vi "NaCTA_configure.vi"() -> ()   [LabVIEW 2020]
uses:
  Instrument drivers/Arduino/ctls_and_globals/Arduino tx msg cluster.ctl
panel:
  in  "a4":dbl=1.0
  in  "a3":dbl=1.0
  in  "Enable USB stream":bool=TRUE
  in  "a2":dbl=1.0
  in  "T0 offset (deg C)":dbl
  in  "P_atmos offset (Pa)":dbl
  in  "Port":refnum<visa-resource-name>
  in  "Get / Set":u8(ring) items=["Get", "Set"]
  in  "a1":dbl=1.0
  in  "a0":dbl=1.0
  out "Read-back":string
  out "Status comment":string
  in  "Address":u8=1
  # "Use this vi to configure the NaCTA 'hot-thermistor' node\nThese settings are retained in EEPROM and recalled on power-up."
  # "PN 05/02/2017"
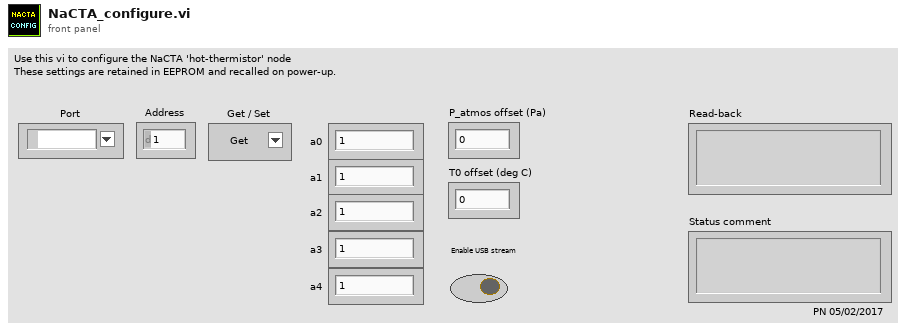
[diagram p1: front panel]
types:
  T1 = typedef "Arduino tx msg cluster.ctl" = cluster{"dest":u8, "A/D/C/I":string, "R/W":string, "chan":u8, "val (float)":sgl}
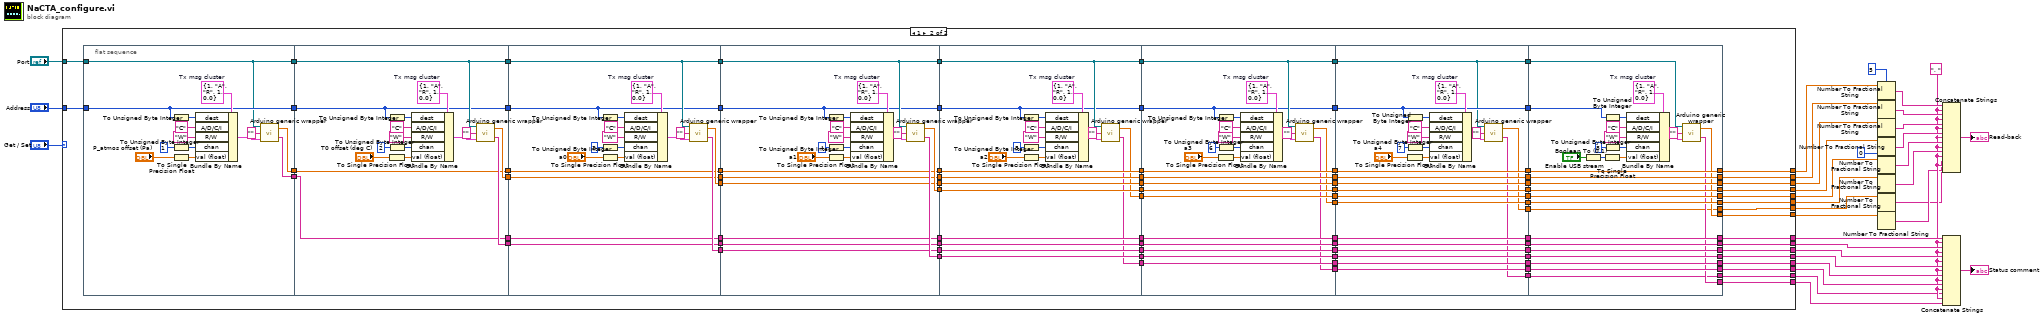
[diagram p0: block diagram]
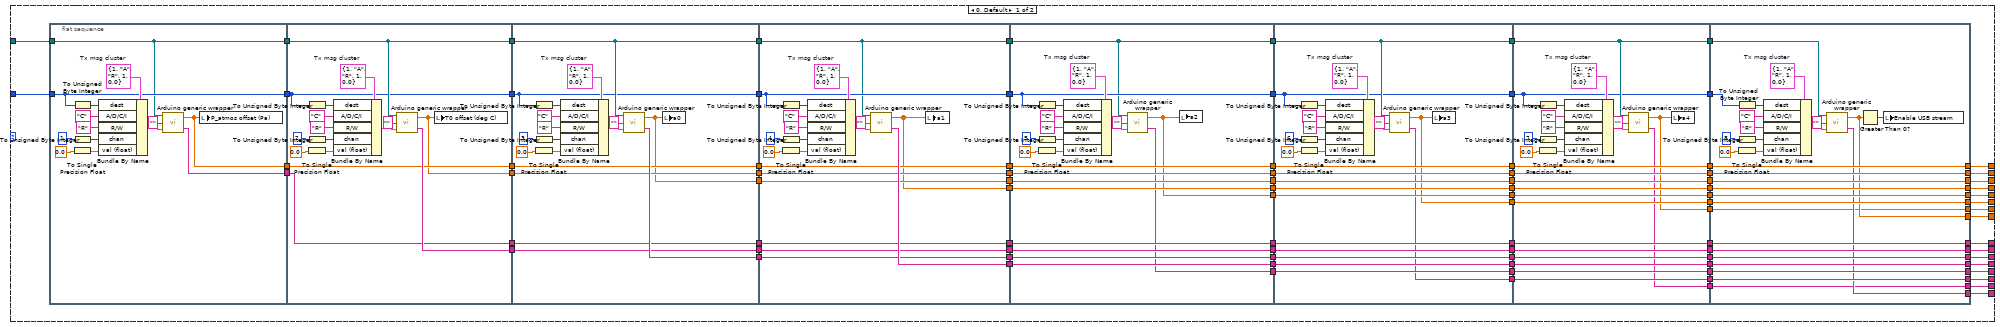
[diagram p2: hidden frame]
diagram:
  w4 = i16 5 ("precision (6)")
  w6 = ", "
  n1 = case shown="1" "Get / Set" {
    tunnel: "Address" -> [w101 w359]
    tunnel: [w93 w358] -> w27
    tunnel: [w97 w357] -> w26
    tunnel: [w98 w356] -> w24
    tunnel: [w94 w355] -> w23
    tunnel: [w95 w354] -> w22
    tunnel: [w96 w353] -> w21
    tunnel: [w99 w352] -> w20
    tunnel: [w100 w351] -> w19
    tunnel: "Port" -> [w102 w350]
    tunnel: [w70 w339] -> w12
    tunnel: [w67 w325] -> w11
    tunnel: [w65 w323] -> w7
    tunnel: [w69 w338] -> w10
    tunnel: [w68 w324] -> w9
    tunnel: [w66 w322] -> w8
    tunnel: [w34 w293] -> w2
    tunnel: [w33 w290] -> w1
    frame 0, Default {
      n2 = flat-sequence {
        tunnel: w101 -> [w126]
        tunnel: w102 -> [w125]
        tunnel: [w125] -> w120
        tunnel: [w126] -> w119
        tunnel: [w122] -> w118
        tunnel: [w124] -> w117
        tunnel: [w142] -> w116
        tunnel: [w141] -> w115
        tunnel: [w140] -> w114
        tunnel: [w136] -> w113
        tunnel: w120 -> [w142]
        tunnel: w119 -> [w141]
        tunnel: w118 -> [w138]
        tunnel: w117 -> [w139]
        tunnel: [w139] -> w112
        tunnel: [w138] -> w111
        tunnel: w116 -> [w160]
        tunnel: [w160] -> w110
        tunnel: w115 -> [w159]
        tunnel: [w159] -> w109
        tunnel: w114 -> [w157]
        tunnel: w113 -> [w155]
        tunnel: [w158] -> w108
        tunnel: [w152] -> w107
        tunnel: [w157] -> w106
        tunnel: [w156] -> w105
        tunnel: w112 -> [w156]
        tunnel: [w155] -> w104
        tunnel: [w154] -> w103
        tunnel: w111 -> [w154]
        tunnel: w110 -> [w171]
        tunnel: w109 -> [w172]
        tunnel: w108 -> [w178]
        tunnel: w107 -> [w179]
        tunnel: w106 -> [w177]
        tunnel: w105 -> [w176]
        tunnel: w104 -> [w175]
        tunnel: w103 -> [w174]
        tunnel: [w180] -> w92
        tunnel: [w170] -> w91
        tunnel: [w179] -> w90
        tunnel: [w178] -> w89
        tunnel: [w177] -> w88
        tunnel: [w176] -> w87
        tunnel: [w175] -> w86
        tunnel: [w174] -> w85
        tunnel: [w172] -> w76
        tunnel: [w171] -> w75
        tunnel: w92 -> [w210]
        tunnel: w91 -> [w209]
        tunnel: w90 -> [w208]
        tunnel: w89 -> [w207]
        tunnel: w88 -> [w206]
        tunnel: w87 -> [w205]
        tunnel: w86 -> [w204]
        tunnel: w85 -> [w203]
        tunnel: [w210] -> w84
        tunnel: [w209] -> w83
        tunnel: [w208] -> w82
        tunnel: [w207] -> w81
        tunnel: [w206] -> w80
        tunnel: [w205] -> w79
        tunnel: [w204] -> w78
        tunnel: [w203] -> w77
        tunnel: w76 -> [w193]
        tunnel: w75 -> [w192]
        tunnel: [w193] -> w74
        tunnel: [w192] -> w73
        tunnel: [w191] -> w72
        tunnel: [w190] -> w71
        tunnel: w84 -> [w234]
        tunnel: w83 -> [w233]
        tunnel: w82 -> [w232]
        tunnel: w81 -> [w231]
        tunnel: w80 -> [w230]
        tunnel: w79 -> [w229]
        tunnel: w78 -> [w228]
        tunnel: w77 -> [w227]
        tunnel: [w234] -> w64
        tunnel: [w233] -> w62
        tunnel: [w232] -> w60
        tunnel: [w231] -> w58
        tunnel: [w230] -> w56
        tunnel: [w229] -> w54
        tunnel: [w228] -> w52
        tunnel: [w227] -> w50
        tunnel: w74 -> [w214]
        tunnel: w73 -> [w215]
        tunnel: [w214] -> w48
        tunnel: [w215] -> w46
        tunnel: w72 -> [w226]
        tunnel: w71 -> [w225]
        tunnel: [w226] -> w44
        tunnel: [w225] -> w42
        tunnel: [w212] -> w40
        tunnel: [w213] -> w38
        tunnel: w64 -> [w260]
        tunnel: [w260] -> w63
        tunnel: w62 -> [w259]
        tunnel: [w259] -> w61
        tunnel: w60 -> [w258]
        tunnel: [w258] -> w59
        tunnel: w58 -> [w257]
        tunnel: [w257] -> w57
        tunnel: w56 -> [w256]
        tunnel: [w256] -> w55
        tunnel: w54 -> [w255]
        tunnel: [w255] -> w53
        tunnel: w52 -> [w254]
        tunnel: [w254] -> w51
        tunnel: w50 -> [w253]
        tunnel: [w253] -> w49
        tunnel: w48 -> [w236]
        tunnel: [w236] -> w47
        tunnel: w46 -> [w239]
        tunnel: [w239] -> w45
        tunnel: w44 -> [w252]
        tunnel: [w252] -> w43
        tunnel: w42 -> [w251]
        tunnel: [w251] -> w41
        tunnel: w40 -> [w250]
        tunnel: [w250] -> w39
        tunnel: w38 -> [w249]
        tunnel: [w249] -> w37
        tunnel: [w238] -> w36
        tunnel: [w237] -> w35
        tunnel: w63 -> [w289]
        tunnel: w61 -> [w288]
        tunnel: w59 -> [w287]
        tunnel: w57 -> [w286]
        tunnel: w55 -> [w285]
        tunnel: w53 -> [w284]
        tunnel: w51 -> [w283]
        tunnel: w49 -> [w282]
        tunnel: w47 -> [w267]
        tunnel: w45 -> [w266]
        tunnel: w43 -> [w281]
        tunnel: w41 -> [w280]
        tunnel: w39 -> [w279]
        tunnel: w37 -> [w278]
        tunnel: [w268] -> w65
        tunnel: [w264] -> w66
        tunnel: [w278] -> w67
        tunnel: [w279] -> w68
        tunnel: [w280] -> w69
        tunnel: [w281] -> w70
        tunnel: [w282] -> w100
        tunnel: [w283] -> w99
        tunnel: [w284] -> w96
        tunnel: [w285] -> w95
        tunnel: [w286] -> w94
        tunnel: [w287] -> w98
        tunnel: [w288] -> w97
        tunnel: [w289] -> w93
        tunnel: w36 -> [w263]
        tunnel: w35 -> [w262]
        tunnel: [w263] -> w34
        tunnel: [w262] -> w33
        frame #0 {
          w134 = T1 {"dest"=1, "A/D/C/I"="A", "R/W"="R", "chan"=1, "val (float)"=0.0}  # Tx msg cluster
          n3 = To Unsigned Byte Integer(number=w126) -> (unsigned 8bit integer=w132:u8)
          n4 = To Unsigned Byte Integer(number=u8 1) -> (unsigned 8bit integer=w133:u8)
          n5 = To Single Precision Float(number=0.0) -> (single precision float=w130:sgl)
          n6 = Bundle By Name(cluster=w134, "dest"=w132, "A/D/C/I"="C" ("A/D"), "R/W"="R", "chan"=w133, "val (float)"=w130) -> (w131:T1)
          n7 = call "Arduino generic wrapper.vi"("Tx msg cluster"=w131, "Channel Name"="", "Port name"=w125) -> ("Scan comment"=w124:string, "Output"=w122:dbl)
          n8 = local write "P_atmos offset (Pa)"(w122) -> ()
        }
        frame #1 {
          w143 = T1 {"dest"=1, "A/D/C/I"="A", "R/W"="R", "chan"=1, "val (float)"=0.0}  # Tx msg cluster
          n9 = To Unsigned Byte Integer(number=w141) -> (unsigned 8bit integer=w145:u8)
          n10 = To Unsigned Byte Integer(number=u8 2) -> (unsigned 8bit integer=w144:u8)
          n11 = To Single Precision Float(number=0.0) -> (single precision float=w147:sgl)
          n12 = Bundle By Name(cluster=w143, "dest"=w145, "A/D/C/I"="C" ("A/D"), "R/W"="R", "chan"=w144, "val (float)"=w147) -> (w146:T1)
          n13 = call "Arduino generic wrapper.vi"("Tx msg cluster"=w146, "Channel Name"="", "Port name"=w142) -> ("Scan comment"=w140:string, "Output"=w136:dbl)
          n14 = local write "T0 offset (deg C)"(w136) -> ()
        }
        frame #2 {
          w168 = T1 {"dest"=1, "A/D/C/I"="A", "R/W"="R", "chan"=1, "val (float)"=0.0}  # Tx msg cluster
          n15 = To Unsigned Byte Integer(number=w159) -> (unsigned 8bit integer=w166:u8)
          n16 = To Unsigned Byte Integer(number=u8 3) -> (unsigned 8bit integer=w167:u8)
          n17 = To Single Precision Float(number=0.0) -> (single precision float=w164:sgl)
          n18 = Bundle By Name(cluster=w168, "dest"=w166, "A/D/C/I"="C" ("A/D"), "R/W"="R", "chan"=w167, "val (float)"=w164) -> (w165:T1)
          n19 = call "Arduino generic wrapper.vi"("Tx msg cluster"=w165, "Channel Name"="", "Port name"=w160) -> ("Scan comment"=w158:string, "Output"=w152:dbl)
          n20 = local write "a0"(w152) -> ()
        }
        frame #3 {
          w187 = T1 {"dest"=1, "A/D/C/I"="A", "R/W"="R", "chan"=1, "val (float)"=0.0}  # Tx msg cluster
          n21 = To Unsigned Byte Integer(number=w172) -> (unsigned 8bit integer=w181:u8)
          n22 = To Unsigned Byte Integer(number=u8 4) -> (unsigned 8bit integer=w182:u8)
          n23 = To Single Precision Float(number=0.0) -> (single precision float=w184:sgl)
          n24 = Bundle By Name(cluster=w187, "dest"=w181, "A/D/C/I"="C" ("A/D"), "R/W"="R", "chan"=w182, "val (float)"=w184) -> (w183:T1)
          n25 = call "Arduino generic wrapper.vi"("Tx msg cluster"=w183, "Channel Name"="", "Port name"=w171) -> ("Scan comment"=w180:string, "Output"=w170:dbl)
          n26 = local write "a1"(w170) -> ()
        }
        frame #4 {
          w195 = T1 {"dest"=1, "A/D/C/I"="A", "R/W"="R", "chan"=1, "val (float)"=0.0}  # Tx msg cluster
          n27 = To Unsigned Byte Integer(number=w193) -> (unsigned 8bit integer=w201:u8)
          n28 = To Unsigned Byte Integer(number=u8 5) -> (unsigned 8bit integer=w200:u8)
          n29 = To Single Precision Float(number=0.0) -> (single precision float=w198:sgl)
          n30 = Bundle By Name(cluster=w195, "dest"=w201, "A/D/C/I"="C" ("A/D"), "R/W"="R", "chan"=w200, "val (float)"=w198) -> (w199:T1)
          n31 = call "Arduino generic wrapper.vi"("Tx msg cluster"=w199, "Channel Name"="", "Port name"=w192) -> ("Scan comment"=w191:string, "Output"=w190:dbl)
          n32 = local write "a2"(w190) -> ()
        }
        frame #5 {
          w223 = T1 {"dest"=1, "A/D/C/I"="A", "R/W"="R", "chan"=1, "val (float)"=0.0}  # Tx msg cluster
          n33 = To Unsigned Byte Integer(number=w214) -> (unsigned 8bit integer=w217:u8)
          n34 = To Unsigned Byte Integer(number=u8 6) -> (unsigned 8bit integer=w218:u8)
          n35 = To Single Precision Float(number=0.0) -> (single precision float=w220:sgl)
          n36 = Bundle By Name(cluster=w223, "dest"=w217, "A/D/C/I"="C" ("A/D"), "R/W"="R", "chan"=w218, "val (float)"=w220) -> (w219:T1)
          n37 = call "Arduino generic wrapper.vi"("Tx msg cluster"=w219, "Channel Name"="", "Port name"=w215) -> ("Scan comment"=w213:string, "Output"=w212:dbl)
          n38 = local write "a3"(w212) -> ()
        }
        frame #6 {
          w241 = T1 {"dest"=1, "A/D/C/I"="A", "R/W"="R", "chan"=1, "val (float)"=0.0}  # Tx msg cluster
          n39 = To Unsigned Byte Integer(number=w236) -> (unsigned 8bit integer=w247:u8)
          n40 = To Unsigned Byte Integer(number=u8 7) -> (unsigned 8bit integer=w246:u8)
          n41 = To Single Precision Float(number=0.0) -> (single precision float=w244:sgl)
          n42 = Bundle By Name(cluster=w241, "dest"=w247, "A/D/C/I"="C" ("A/D"), "R/W"="R", "chan"=w246, "val (float)"=w244) -> (w245:T1)
          n43 = call "Arduino generic wrapper.vi"("Tx msg cluster"=w245, "Channel Name"="", "Port name"=w239) -> ("Scan comment"=w237:string, "Output"=w238:dbl)
          n44 = local write "a4"(w238) -> ()
        }
        frame #7 {
          w270 = T1 {"dest"=1, "A/D/C/I"="A", "R/W"="R", "chan"=1, "val (float)"=0.0}  # Tx msg cluster
          n45 = To Unsigned Byte Integer(number=w267) -> (unsigned 8bit integer=w276:u8)
          n46 = To Unsigned Byte Integer(number=u8 8) -> (unsigned 8bit integer=w275:u8)
          n47 = To Single Precision Float(number=0.0) -> (single precision float=w273:sgl)
          n48 = Bundle By Name(cluster=w270, "dest"=w276, "A/D/C/I"="C" ("A/D"), "R/W"="R", "chan"=w275, "val (float)"=w273) -> (w274:T1)
          n49 = call "Arduino generic wrapper.vi"("Tx msg cluster"=w274, "Channel Name"="", "Port name"=w266) -> ("Scan comment"=w268:string, "Output"=w264:dbl)
          n50 = Greater Than 0?(x=w264) -> (x > 0?=w265:bool)
          n51 = local write "Enable USB stream"(w265) -> ()
        }
      }
    }
    frame 1 {
      n52 = flat-sequence {
        tunnel: w359 -> [w383]
        tunnel: w350 -> [w382]
        tunnel: [w382] -> w377
        tunnel: [w383] -> w376
        tunnel: [w381] -> w375
        tunnel: [w380] -> w374
        tunnel: [w399] -> w373
        tunnel: [w398] -> w372
        tunnel: [w397] -> w371
        tunnel: [w396] -> w370
        tunnel: w377 -> [w399]
        tunnel: w376 -> [w398]
        tunnel: w375 -> [w394]
        tunnel: w374 -> [w395]
        tunnel: [w395] -> w369
        tunnel: [w394] -> w368
        tunnel: w373 -> [w417]
        tunnel: [w417] -> w367
        tunnel: w372 -> [w416]
        tunnel: [w416] -> w366
        tunnel: w371 -> [w413]
        tunnel: w370 -> [w411]
        tunnel: [w415] -> w365
        tunnel: [w414] -> w364
        tunnel: [w413] -> w363
        tunnel: [w412] -> w362
        tunnel: w369 -> [w412]
        tunnel: [w411] -> w361
        tunnel: [w410] -> w360
        tunnel: w368 -> [w410]
        tunnel: w367 -> [w429]
        tunnel: w366 -> [w428]
        tunnel: w365 -> [w434]
        tunnel: w364 -> [w435]
        tunnel: w363 -> [w433]
        tunnel: w362 -> [w432]
        tunnel: w361 -> [w431]
        tunnel: w360 -> [w430]
        tunnel: [w437] -> w349
        tunnel: [w436] -> w348
        tunnel: [w435] -> w347
        tunnel: [w434] -> w346
        tunnel: [w433] -> w345
        tunnel: [w432] -> w344
        tunnel: [w431] -> w343
        tunnel: [w430] -> w342
        tunnel: [w429] -> w341
        tunnel: [w428] -> w340
        tunnel: w349 -> [w467]
        tunnel: w348 -> [w466]
        tunnel: w347 -> [w465]
        tunnel: w346 -> [w464]
        tunnel: w345 -> [w463]
        tunnel: w344 -> [w462]
        tunnel: w343 -> [w461]
        tunnel: w342 -> [w460]
        tunnel: w341 -> [w449]
        tunnel: w340 -> [w448]
        tunnel: [w467] -> w337
        tunnel: [w466] -> w336
        tunnel: [w465] -> w335
        tunnel: [w464] -> w334
        tunnel: [w463] -> w333
        tunnel: [w462] -> w332
        tunnel: [w461] -> w331
        tunnel: [w460] -> w330
        tunnel: [w451] -> w329
        tunnel: [w450] -> w328
        tunnel: [w449] -> w327
        tunnel: [w448] -> w326
        tunnel: w337 -> [w491]
        tunnel: w336 -> [w490]
        tunnel: w335 -> [w489]
        tunnel: w334 -> [w488]
        tunnel: w333 -> [w487]
        tunnel: w332 -> [w486]
        tunnel: w331 -> [w485]
        tunnel: w330 -> [w484]
        tunnel: w329 -> [w483]
        tunnel: w328 -> [w482]
        tunnel: w327 -> [w471]
        tunnel: w326 -> [w470]
        tunnel: [w491] -> w321
        tunnel: [w490] -> w319
        tunnel: [w489] -> w317
        tunnel: [w488] -> w315
        tunnel: [w487] -> w313
        tunnel: [w486] -> w311
        tunnel: [w485] -> w309
        tunnel: [w484] -> w307
        tunnel: [w483] -> w305
        tunnel: [w482] -> w303
        tunnel: [w473] -> w301
        tunnel: [w472] -> w299
        tunnel: [w471] -> w297
        tunnel: [w470] -> w295
        tunnel: w321 -> [w517]
        tunnel: [w517] -> w320
        tunnel: w319 -> [w516]
        tunnel: [w516] -> w318
        tunnel: w317 -> [w515]
        tunnel: [w515] -> w316
        tunnel: w315 -> [w514]
        tunnel: [w514] -> w314
        tunnel: w313 -> [w513]
        tunnel: [w513] -> w312
        tunnel: w311 -> [w512]
        tunnel: [w512] -> w310
        tunnel: w309 -> [w511]
        tunnel: [w511] -> w308
        tunnel: w307 -> [w510]
        tunnel: [w510] -> w306
        tunnel: w305 -> [w509]
        tunnel: [w509] -> w304
        tunnel: w303 -> [w508]
        tunnel: [w508] -> w302
        tunnel: w301 -> [w507]
        tunnel: [w507] -> w300
        tunnel: w299 -> [w506]
        tunnel: [w506] -> w298
        tunnel: w297 -> [w495]
        tunnel: [w495] -> w296
        tunnel: w295 -> [w496]
        tunnel: [w496] -> w294
        tunnel: [w494] -> w292
        tunnel: [w493] -> w291
        tunnel: w320 -> [w546]
        tunnel: w318 -> [w545]
        tunnel: w316 -> [w544]
        tunnel: w314 -> [w543]
        tunnel: w312 -> [w542]
        tunnel: w310 -> [w541]
        tunnel: w308 -> [w540]
        tunnel: w306 -> [w539]
        tunnel: w304 -> [w538]
        tunnel: w302 -> [w537]
        tunnel: w300 -> [w536]
        tunnel: w298 -> [w535]
        tunnel: w296 -> [w523]
        tunnel: w294 -> [w524]
        tunnel: [w525] -> w322
        tunnel: [w526] -> w323
        tunnel: [w535] -> w324
        tunnel: [w536] -> w325
        tunnel: [w537] -> w338
        tunnel: [w538] -> w339
        tunnel: [w539] -> w351
        tunnel: [w540] -> w352
        tunnel: [w541] -> w353
        tunnel: [w542] -> w354
        tunnel: [w543] -> w355
        tunnel: [w544] -> w356
        tunnel: [w545] -> w357
        tunnel: [w546] -> w358
        tunnel: [w520] -> w293
        tunnel: w292 -> [w520]
        tunnel: w291 -> [w519]
        tunnel: [w519] -> w290
        frame #0 {
          w391 = T1 {"dest"=1, "A/D/C/I"="A", "R/W"="R", "chan"=1, "val (float)"=0.0}  # Tx msg cluster
          n53 = To Unsigned Byte Integer(number=w383) -> (unsigned 8bit integer=w389:u8)
          n54 = To Unsigned Byte Integer(number=u8 1) -> (unsigned 8bit integer=w390:u8)
          n55 = To Single Precision Float(number="P_atmos offset (Pa)") -> (single precision float=w387:sgl)
          n56 = Bundle By Name(cluster=w391, "dest"=w389, "A/D/C/I"="C" ("A/D"), "R/W"="W", "chan"=w390, "val (float)"=w387) -> (w388:T1)
          n57 = call "Arduino generic wrapper.vi"("Tx msg cluster"=w388, "Channel Name"="", "Port name"=w382) -> ("Scan comment"=w380:string, "Output"=w381:dbl)
        }
        frame #1 {
          w400 = T1 {"dest"=1, "A/D/C/I"="A", "R/W"="R", "chan"=1, "val (float)"=0.0}  # Tx msg cluster
          n58 = To Unsigned Byte Integer(number=w398) -> (unsigned 8bit integer=w402:u8)
          n59 = To Unsigned Byte Integer(number=u8 2) -> (unsigned 8bit integer=w401:u8)
          n60 = To Single Precision Float(number="T0 offset (deg C)") -> (single precision float=w404:sgl)
          n61 = Bundle By Name(cluster=w400, "dest"=w402, "A/D/C/I"="C" ("A/D"), "R/W"="W", "chan"=w401, "val (float)"=w404) -> (w403:T1)
          n62 = call "Arduino generic wrapper.vi"("Tx msg cluster"=w403, "Channel Name"="", "Port name"=w399) -> ("Scan comment"=w397:string, "Output"=w396:dbl)
        }
        frame #2 {
          w425 = T1 {"dest"=1, "A/D/C/I"="A", "R/W"="R", "chan"=1, "val (float)"=0.0}  # Tx msg cluster
          n63 = To Unsigned Byte Integer(number=w416) -> (unsigned 8bit integer=w423:u8)
          n64 = To Unsigned Byte Integer(number=u8 3) -> (unsigned 8bit integer=w424:u8)
          n65 = To Single Precision Float(number="a0") -> (single precision float=w421:sgl)
          n66 = Bundle By Name(cluster=w425, "dest"=w423, "A/D/C/I"="C" ("A/D"), "R/W"="W", "chan"=w424, "val (float)"=w421) -> (w422:T1)
          n67 = call "Arduino generic wrapper.vi"("Tx msg cluster"=w422, "Channel Name"="", "Port name"=w417) -> ("Scan comment"=w415:string, "Output"=w414:dbl)
        }
        frame #3 {
          w444 = T1 {"dest"=1, "A/D/C/I"="A", "R/W"="R", "chan"=1, "val (float)"=0.0}  # Tx msg cluster
          n68 = To Unsigned Byte Integer(number=w428) -> (unsigned 8bit integer=w438:u8)
          n69 = To Unsigned Byte Integer(number=u8 4) -> (unsigned 8bit integer=w439:u8)
          n70 = To Single Precision Float(number="a1") -> (single precision float=w441:sgl)
          n71 = Bundle By Name(cluster=w444, "dest"=w438, "A/D/C/I"="C" ("A/D"), "R/W"="W", "chan"=w439, "val (float)"=w441) -> (w440:T1)
          n72 = call "Arduino generic wrapper.vi"("Tx msg cluster"=w440, "Channel Name"="", "Port name"=w429) -> ("Scan comment"=w437:string, "Output"=w436:dbl)
        }
        frame #4 {
          w453 = T1 {"dest"=1, "A/D/C/I"="A", "R/W"="R", "chan"=1, "val (float)"=0.0}  # Tx msg cluster
          n73 = To Unsigned Byte Integer(number=w448) -> (unsigned 8bit integer=w459:u8)
          n74 = To Unsigned Byte Integer(number=u8 5) -> (unsigned 8bit integer=w458:u8)
          n75 = To Single Precision Float(number="a2") -> (single precision float=w456:sgl)
          n76 = Bundle By Name(cluster=w453, "dest"=w459, "A/D/C/I"="C" ("A/D"), "R/W"="W", "chan"=w458, "val (float)"=w456) -> (w457:T1)
          n77 = call "Arduino generic wrapper.vi"("Tx msg cluster"=w457, "Channel Name"="", "Port name"=w449) -> ("Scan comment"=w451:string, "Output"=w450:dbl)
        }
        frame #5 {
          w480 = T1 {"dest"=1, "A/D/C/I"="A", "R/W"="R", "chan"=1, "val (float)"=0.0}  # Tx msg cluster
          n78 = To Unsigned Byte Integer(number=w470) -> (unsigned 8bit integer=w474:u8)
          n79 = To Unsigned Byte Integer(number=u8 6) -> (unsigned 8bit integer=w475:u8)
          n80 = To Single Precision Float(number="a3") -> (single precision float=w477:sgl)
          n81 = Bundle By Name(cluster=w480, "dest"=w474, "A/D/C/I"="C" ("A/D"), "R/W"="W", "chan"=w475, "val (float)"=w477) -> (w476:T1)
          n82 = call "Arduino generic wrapper.vi"("Tx msg cluster"=w476, "Channel Name"="", "Port name"=w471) -> ("Scan comment"=w473:string, "Output"=w472:dbl)
        }
        frame #6 {
          w499 = T1 {"dest"=1, "A/D/C/I"="A", "R/W"="R", "chan"=1, "val (float)"=0.0}  # Tx msg cluster
          n83 = To Unsigned Byte Integer(number=w496) -> (unsigned 8bit integer=w505:u8)
          n84 = To Unsigned Byte Integer(number=u8 7) -> (unsigned 8bit integer=w504:u8)
          n85 = To Single Precision Float(number="a4") -> (single precision float=w502:sgl)
          n86 = Bundle By Name(cluster=w499, "dest"=w505, "A/D/C/I"="C" ("A/D"), "R/W"="W", "chan"=w504, "val (float)"=w502) -> (w503:T1)
          n87 = call "Arduino generic wrapper.vi"("Tx msg cluster"=w503, "Channel Name"="", "Port name"=w495) -> ("Scan comment"=w493:string, "Output"=w494:dbl)
        }
        frame #7 {
          w528 = T1 {"dest"=1, "A/D/C/I"="A", "R/W"="R", "chan"=1, "val (float)"=0.0}  # Tx msg cluster
          n88 = Boolean To (0,1)(Boolean="Enable USB stream") -> (0, 1=w522:i16)
          n89 = To Unsigned Byte Integer(number=w524) -> (unsigned 8bit integer=w534:u8)
          n90 = To Unsigned Byte Integer(number=u8 8) -> (unsigned 8bit integer=w533:u8)
          n91 = To Single Precision Float(number=w522) -> (single precision float=w531:sgl)
          n92 = Bundle By Name(cluster=w528, "dest"=w534, "A/D/C/I"="C" ("A/D"), "R/W"="W", "chan"=w533, "val (float)"=w531) -> (w532:T1)
          n93 = call "Arduino generic wrapper.vi"("Tx msg cluster"=w532, "Channel Name"="", "Port name"=w523) -> ("Scan comment"=w526:string, "Output"=w525:dbl)
        }
      }
    }
  }
  n94 = Number To Fractional String(number=w19, precision (6)=w4) -> (F-format string=w31:string)  [unwired: 2 in]
  n95 = Number To Fractional String(number=w20, precision (6)=w4) -> (F-format string=w30:string)  [unwired: 2 in]
  n96 = Number To Fractional String(number=w24, precision (6)=w4) -> (F-format string=w18:string)  [unwired: 2 in]
  n97 = Number To Fractional String(number=w26, precision (6)=i16 0) -> (F-format string=w17:string)  [unwired: 2 in]
  n98 = Number To Fractional String(number=w10, precision (6)=w4) -> (F-format string=w14:string)  [unwired: 2 in]
  n99 = Number To Fractional String(number=w9, precision (6)=w4) -> (F-format string=w13:string)  [unwired: 2 in]
  n100 = Number To Fractional String(number=w2, precision (6)=w4) -> (F-format string=w3:string)  [unwired: 2 in]
  n101 = Number To Fractional String(number=w8, precision (6)=w4) -> (F-format string=w5:string)  [unwired: 2 in]
  n102 = Concatenate Strings(w31, w6, w30, w6, w18, w6, w17, w6, w14, w6, w13, w6, w3, w6, w5) -> (→"Read-back":string)
  n103 = Concatenate Strings(w21, w6, w22, w6, w23, w6, w27, w6, w12, w6, w11, w6, w1, w6, w7) -> (→"Status comment":string)
